vi "GenerateXYArmPathPolygon.vi"(2 "PointSpacing (in)":dbl, 3 "MaxRadius (in)":dbl, 4 "End_Y (in)":dbl, 5 "End_X (in)":dbl, 6 "Start_Y (in)":dbl, 7 "Start_X (in)":dbl) -> (0 "Angles":dbl[](array[numeric]), 1 "Radii":dbl[](array[numeric]))   [LabVIEW 2017]
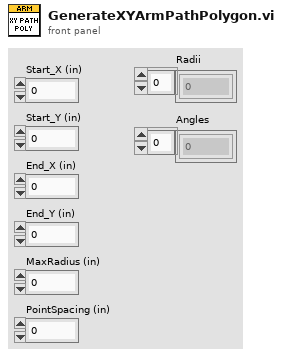
[diagram p1: front panel]
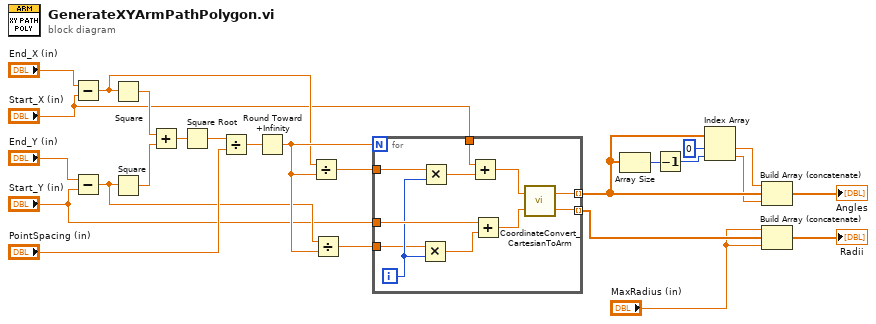
[diagram p0: block diagram]
diagram:
  n1 = Subtract(x="End_X (in)", y="Start_X (in)") -> (x-y=w18:dbl)
  n2 = Subtract(x="End_Y (in)", y="Start_Y (in)") -> (x-y=w17:dbl)
  n3 = Square(x=w18) -> (x^2=w25:dbl)
  n4 = Square(x=w17) -> (x^2=w24:dbl)
  n5 = Add(x=w25, y=w24) -> (x+y=w23:dbl)
  n6 = Square Root(x=w23) -> (sqrt(x)=w22:dbl)
  n7 = Divide(x=w22, y="PointSpacing (in)") -> (x/y=w20:dbl)
  n8 = Round Toward +Infinity(x=w20) -> (ceil(x): smallest int >= x=w19:dbl)
  n9 = Divide(x=w18, y=w19) -> (x/y=w15:dbl)
  n10 = Divide(x=w17, y=w19) -> (x/y=w16:dbl)
  n11 = for {
    N: w19 -> [_]
    tunnel: "Start_X (in)" -> [w36]
    tunnel: "Start_Y (in)" -> [w35]
    tunnel: w16 -> [w31]
    tunnel: w15 -> [w30]
    tunnel: [w27] -> w6 mode=indexing
    tunnel: [w26] -> w10 mode=indexing
    i -> [w33]
    n12 = Multiply(x=w31, y=w33) -> (x*y=w34:dbl)
    n13 = Multiply(x=w30, y=w33) -> (x*y=w32:dbl)
    n14 = Add(x=w36, y=w32) -> (x+y=w28:dbl)
    n15 = Add(x=w35, y=w34) -> (x+y=w29:dbl)
    n16 = call "CoordinateConvert_CartesianToArm.vi"("Y (in)"=w29, "X (in)"=w28) -> ("Radius (in)"=w26:dbl, "Angle (rad)"=w27:dbl)
  }
  n17 = Array Size(array=w6) -> (size(s)=w5:i32)
  n18 = Decrement(x=w5) -> (x-1=w4:i32)
  n19 = Index Array(array=w6, index #1=0 ("index"), index #2=w4) -> (element #1=w3:dbl, element #2=w2:dbl)
  n20 = Build Array (concatenate)(w3, w6, w2) -> (→"Angles":dbl[])
  n21 = Build Array (concatenate)("MaxRadius (in)", w10, "MaxRadius (in)") -> (→"Radii":dbl[])
